vi "waveformpreparept1.vi"(8 "Heat Time(units of 1 us)":dbl, 9 "1762 pulse length (units of 1 us)":dbl=50.0) -> (3 "digital waveform out 2":digitalwaveform(waveform)={"t0"=timestamp(0 s since 1904-01-01), "dt"=1e-07, "Y"={"transitions"=[0, 2100, 2200, 2300, 2301, 3851, 3951], "data"=[[1, 1, 1, 0, 0], [1, 0, 1, 0, 0], [1, 0, 0, 0, 0], [0, 0, 0, 0, 0], [0, 0, 0, 0, 1], [0, 0, 0, 0, 0], [0, 1, 1, 0, 0]]}, "error"={"status"=FALSE, "code"=37421928, "source"=""}})   [LabVIEW 2012]
uses:
  <vilib>/Waveform/DWDTOps.llb/Digital Pattern Generator (Single Value).vi
  <vilib>/Waveform/DWDTOps.llb/DWDT Append Digital Samples.vi
panel:
  out "Mixed Signal Graph":digitalwaveform(graph)={"t0"=timestamp(0 s since 1904-01-01), "dt"=1e-07, "Y"={"transitions"=[0, 2100, 2200, 2300, 2301, 3851, 3951], "data"=[[1, 1, 1, 0, 0], [1, 0, 1, 0, 0], [1, 0, 0, 0, 0], [0, 0, 0, 0, 0], [0, 0, 0, 0, 1], [0, 0, 0, 0, 0], [0, 1, 1, 0, 0]]}, "error"={"status"=FALSE, "code"=37421928, "source"=""}}
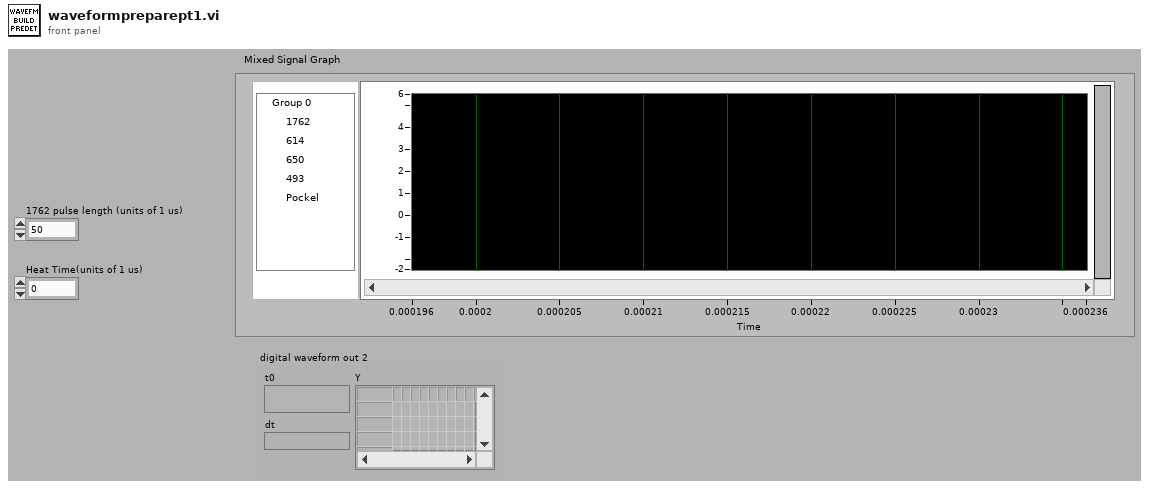
[diagram p1: front panel]
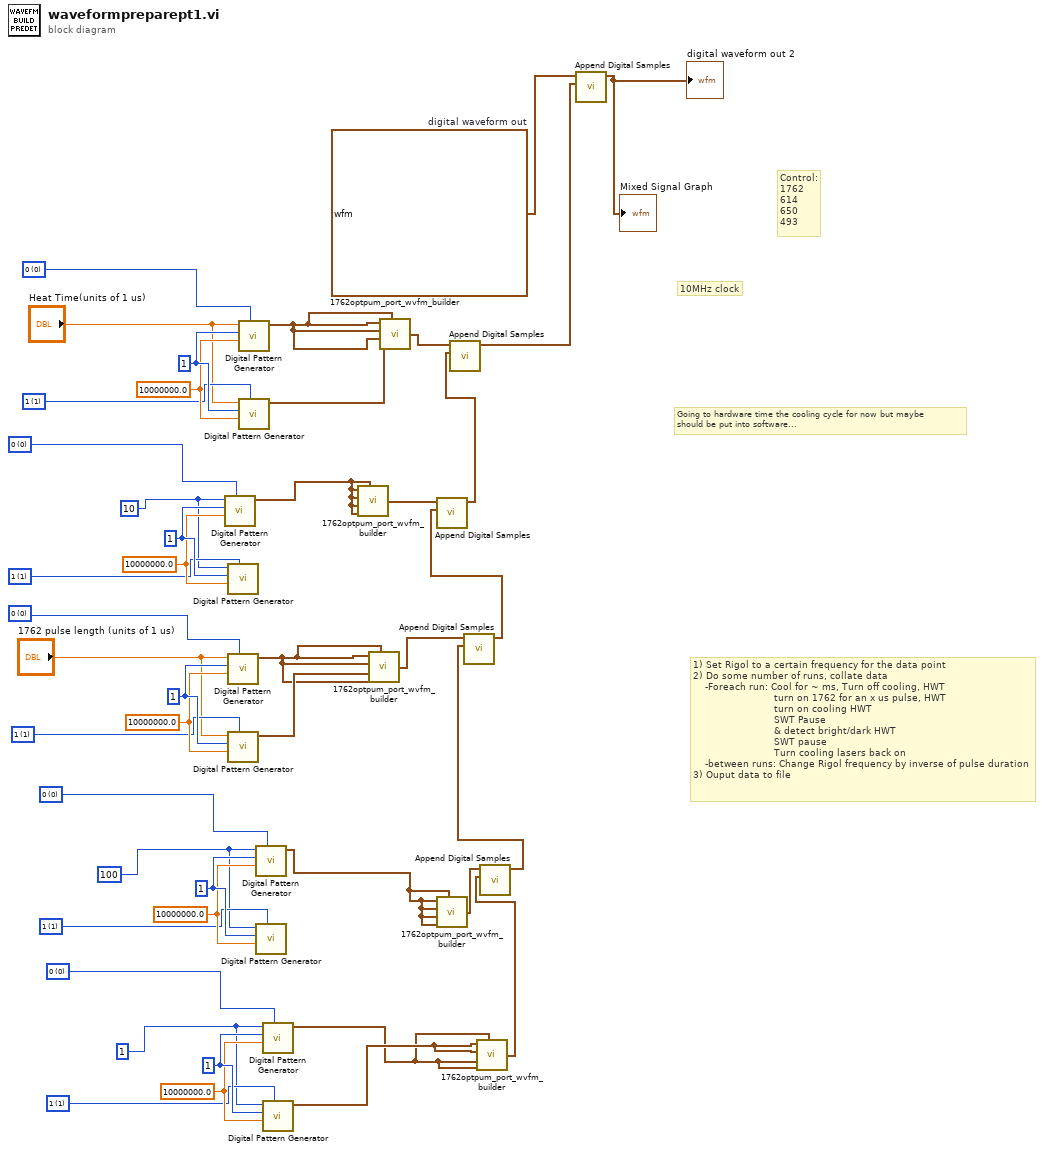
[diagram p0: block diagram]
diagram:
  w5 = u32 10 ("number of samples")
  w9 = u8 0 items=["0", "1", "Z", "L", "H", "X", "T", "V"] ("value")
  w8 = u32 1 ("number of signals")
  w6 = u8 1 items=["0", "1", "Z", "L", "H", "X", "T", "V"] ("value")
  w7 = 10000000.0 ("rate")
  w18 = u8 0 items=["0", "1", "Z", "L", "H", "X", "T", "V"] ("value")
  w17 = u32 1 ("number of signals")
  w15 = u8 1 items=["0", "1", "Z", "L", "H", "X", "T", "V"] ("value")
  w16 = 10000000.0 ("rate")
  w28 = u32 1 ("number of samples")
  w32 = u8 0 items=["0", "1", "Z", "L", "H", "X", "T", "V"] ("value")
  w31 = u32 1 ("number of signals")
  w29 = u8 1 items=["0", "1", "Z", "L", "H", "X", "T", "V"] ("value")
  w30 = 10000000.0 ("rate")
  w33 = u32 100 ("number of samples")
  w37 = u8 0 items=["0", "1", "Z", "L", "H", "X", "T", "V"] ("value")
  w36 = u32 1 ("number of signals")
  w34 = u8 1 items=["0", "1", "Z", "L", "H", "X", "T", "V"] ("value")
  w35 = 10000000.0 ("rate")
  w44 = u8 0 items=["0", "1", "Z", "L", "H", "X", "T", "V"] ("value")
  w43 = u32 1 ("number of signals")
  w41 = u8 1 items=["0", "1", "Z", "L", "H", "X", "T", "V"] ("value")
  w42 = 10000000.0 ("rate")
  w38 = digitalwaveform {"t0"=timestamp(0 s since 1904-01-01), "dt"=1e-07, "Y"={"transitions"=[0, 2100, 2200, 2300], "data"=[[1, 1, 1, 0, 0], [1, 0, 1, 0, 0], [1, 0, 0, 0, 0], [0, 0, 0, 0, 0]]}, "error"={"status"=FALSE, "code"=37421928, "source"=""}}  # digital waveform out
  # "Going to hardware time the cooling cycle for now but maybe\nshould be put into software..."
  # "10MHz clock"
  # "Control:\n1762\n614\n650\n493"
  # "1) Set Rigol to a certain frequency for the data point\n2) Do some number of runs, collate data\n    -Foreach run: Cool for ~ ms, Turn off cooling, HWT\n                           turn on 1762 for an x us pulse, HWT\n                           turn on cooling HWT\n                           SWT Pause\n                           & detect bright/dark HWT\n                           SWT pause\n                           Turn cooling lasers back on \n    -between runs: Change Rigol frequency by inverse of pulse duration\n3) Ouput data to file"
  n1 = call-poly <vilib>:"Digital Pattern Generator.vi"("value"=w9, "sample rate"=w7, "number of signals"=w8, "number of samples"=w5) -> ("digital waveform"=w4:digitalwaveform)  [unwired: 6 in, 1 out]
  n2 = call-poly <vilib>:"Digital Pattern Generator.vi"("value"=w6, "sample rate"=w7, "number of signals"=w8, "number of samples"=w5) -> ()  [unwired: 6 in, 2 out]
  n3 = call-poly <vilib>:"Digital Pattern Generator.vi"("value"=w44, "sample rate"=w42, "number of signals"=w43, "number of samples"="1762 pulse length (units of 1 us)") -> ("digital waveform"=w20:digitalwaveform)  [unwired: 6 in, 1 out]
  n4 = call-poly <vilib>:"Digital Pattern Generator.vi"("value"=w41, "sample rate"=w42, "number of signals"=w43, "number of samples"="1762 pulse length (units of 1 us)") -> ("digital waveform"=w21:digitalwaveform)  [unwired: 6 in, 1 out]
  n5 = call-poly <vilib>:"Digital Pattern Generator.vi"("value"=w18, "sample rate"=w16, "number of signals"=w17, "number of samples"="Heat Time(units of 1 us)") -> ("digital waveform"=w13:digitalwaveform)  [unwired: 6 in, 1 out]
  n6 = call-poly <vilib>:"Digital Pattern Generator.vi"("value"=w15, "sample rate"=w16, "number of signals"=w17, "number of samples"="Heat Time(units of 1 us)") -> ("digital waveform"=w10:digitalwaveform)  [unwired: 6 in, 1 out]
  n7 = call-poly <vilib>:"Digital Pattern Generator.vi"("value"=w37, "sample rate"=w35, "number of signals"=w36, "number of samples"=w33) -> ("digital waveform"=w19:digitalwaveform)  [unwired: 6 in, 1 out]
  n8 = call-poly <vilib>:"Digital Pattern Generator.vi"("value"=w34, "sample rate"=w35, "number of signals"=w36, "number of samples"=w33) -> ()  [unwired: 6 in, 2 out]
  n9 = call-poly <vilib>:"Digital Pattern Generator.vi"("value"=w32, "sample rate"=w30, "number of signals"=w31, "number of samples"=w28) -> ("digital waveform"=w23:digitalwaveform)  [unwired: 6 in, 1 out]
  n10 = call-poly <vilib>:"Digital Pattern Generator.vi"("value"=w29, "sample rate"=w30, "number of signals"=w31, "number of samples"=w28) -> ("digital waveform"=w24:digitalwaveform)  [unwired: 6 in, 1 out]
  n11 = call "1762optpum_port_wvfm_builder.vi"("493"=w4, "650"=w4, "1762"=w4, "614"=w4, "pockel"=w4) -> ("out"=w1:digitalwaveform)
  n12 = call "1762optpum_port_wvfm_builder.vi"("493"=w20, "650"=w20, "1762"=w21, "614"=w20, "pockel"=w20) -> ("out"=w26:digitalwaveform)
  n13 = call "1762optpum_port_wvfm_builder.vi"("493"=w13, "650"=w13, "1762"=w13, "614"=w10, "pockel"=w13) -> ("out"=w12:digitalwaveform)
  n14 = call "1762optpum_port_wvfm_builder.vi"("493"=w19, "650"=w19, "1762"=w19, "614"=w19, "pockel"=w19) -> ("out"=w25:digitalwaveform)
  n15 = call "1762optpum_port_wvfm_builder.vi"("493"=w24, "650"=w24, "1762"=w23, "614"=w23, "pockel"=w23) -> ("out"=w22:digitalwaveform)
  n16 = call-poly <vilib>:"Append Digital Samples.vi"("digital waveform B"=w22, "digital waveform A"=w25) -> ("digital waveform out"=w27:digitalwaveform)  [unwired: 8 in, 1 out]
  n17 = call-poly <vilib>:"Append Digital Samples.vi"("digital waveform B"=w27, "digital waveform A"=w26) -> ("digital waveform out"=w2:digitalwaveform)  [unwired: 8 in, 1 out]
  n18 = call-poly <vilib>:"Append Digital Samples.vi"("digital waveform B"=w2, "digital waveform A"=w1) -> ("digital waveform out"=w3:digitalwaveform)  [unwired: 8 in, 1 out]
  n19 = call-poly <vilib>:"Append Digital Samples.vi"("digital waveform B"=w3, "digital waveform A"=w12) -> ("digital waveform out"=w11:digitalwaveform)  [unwired: 8 in, 1 out]
  n20 = call-poly <vilib>:"Append Digital Samples.vi"("digital waveform B"=w11, "digital waveform A"=w38) -> ("digital waveform out"=→"Mixed Signal Graph" →"digital waveform out 2":digitalwaveform)  [unwired: 8 in, 1 out]
